vi "Calculate Attack Points.vi"(7 "Move Map":i32[][](array[numeric]), 8 "Team Index":i32, 9 "Max Atack Points":i32=4, 11 "Danger Map":i32[][](array[numeric])) -> (2 "Danger Columns Out":i32[](array[numeric]), 3 "Danger Rows Out":i32[](array[numeric]), 5 "Scores Out":i32[](array[numeric]))   [LabVIEW 2017, in "AntFarm_MB.lvclass"]
uses:
  AntFarm_MB.lvclass
panel:
  in  "Distance Threshold":dbl=2.9
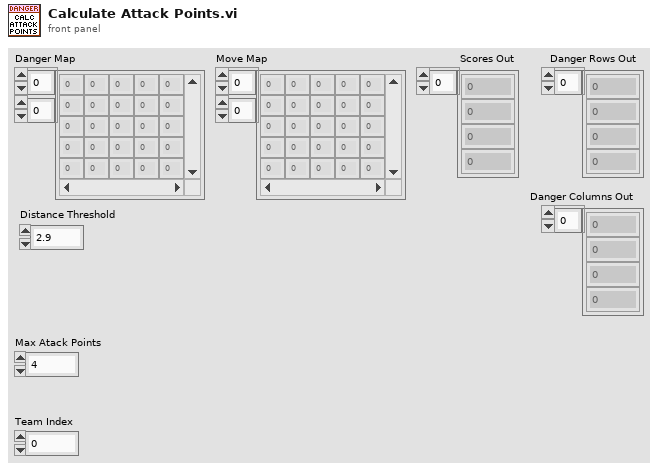
[diagram p1: front panel]
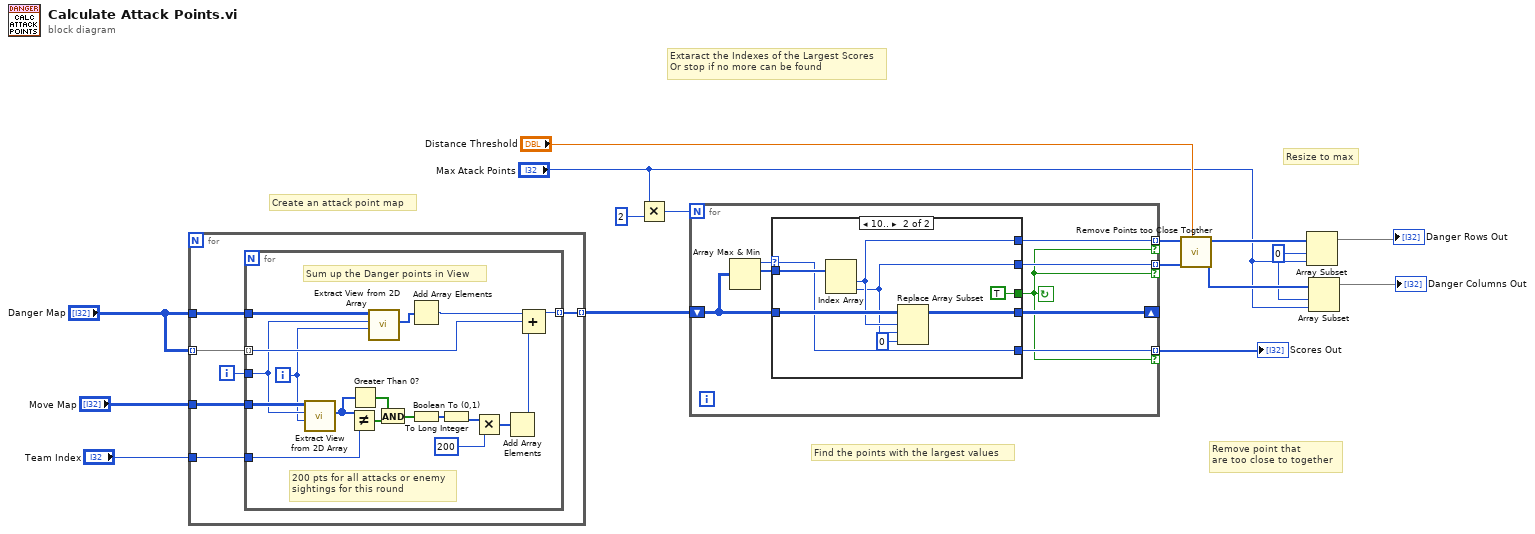
[diagram p0: block diagram]
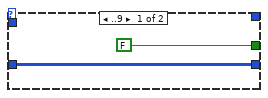
[diagram p2: hidden frame]
diagram:
  w1 = 0 ("index")
  # "Resize to max"
  # "Remove point that\nare too close to together"
  # "Find the points with the largest values"
  # "Create an attack point map"
  # "Extaract the Indexes of the Largest Scores\nOr stop if no more can be found"
  n1 = for {
    tunnel: "Danger Map" -> [w22] mode=indexing
    tunnel: "Danger Map" -> [w21]
    tunnel: [w19] -> w15 mode=indexing
    tunnel: "Move Map" -> [w18]
    tunnel: "Team Index" -> [w17]
    i -> [w20]
    n2 = for {
      tunnel: w22 -> [w37] mode=indexing
      tunnel: w21 -> [w40]
      tunnel: w20 -> [w30]
      tunnel: [w38] -> w19 mode=indexing
      tunnel: w18 -> [w33]
      tunnel: w17 -> [w35]
      i -> [w29]
      # "Sum up the Danger points in View"
      # "200 pts for all attacks or enemy\nsightings for this round"
      n3 = call "Extract View from 2D Array.vi"("Column"=w29, "Row"=w30, "Board Array"=w33) -> ("View Out"=w32:i32[])  [unwired: 7 in, 1 out]
      n4 = Not Equal?(x=w32, y=w35) -> (x != y?=w34:bool[])
      n5 = Greater Than 0?(x=w32) -> (x > 0?=w31:bool[])
      n6 = call "Extract View from 2D Array.vi"("Column"=w29, "Row"=w30, "Board Array"=w40) -> ("View Out"=w36:i32[])  [unwired: 7 in, 1 out]
      n7 = And(x=w31, y=w34) -> (x .and. y?=w28:bool[])
      n8 = Add Array Elements(numeric array=w36) -> (sum=w39:i32)
      n9 = Boolean To (0,1)(Boolean=w28) -> (0, 1=w27:i16[])
      n10 = To Long Integer(number=w27) -> (32bit integer=w26:i32[])
      n11 = Multiply(x=w26, y=200 ("Team Index 2")) -> (x*y=w24:i32[])
      n12 = Add Array Elements(numeric array=w24) -> (sum=w23:i32)
      n13 = Compound Arithmetic op=ADD(w39, w37, w23) -> (w38:i32)
    }
  }
  n14 = Multiply(x="Max Atack Points", y=2) -> (x*y=w11:i32)
  n15 = for {
    N: w11 -> [_]
    shift-right: [w46] -> _
    shift-left: w15 -> [w47]
    tunnel: [w44] -> w14 mode=indexing if=w41
    tunnel: [w43] -> w9 mode=indexing if=w41
    tunnel: [w42] -> w8 mode=indexing if=w41
    stop <- w41 continue-if-true
    n16 = Array Max & Min(array=w47) -> (max value=w48:i32, max index (indices)=w45:i32[])  [unwired: 2 out]
    n17 = case shown="10.." w48 {
      selector: w48 -> [_ w51]
      tunnel: w47 -> [w50 w56]
      tunnel: [w50 w55] -> w46
      tunnel: [FALSE TRUE] -> w41
      tunnel: w45 -> [_ w58]
      tunnel: [_ w51] -> w44
      tunnel: [_ w54] -> w43
      tunnel: [_ w53] -> w42
      frame ..9 {
      }
      frame 10.. {
        n18 = Index Array(array=w58) -> (element #1=w54:i32, element #2=w53:i32)  [unwired: 2 in]
        n19 = Replace Array Subset(array=w56, new element=0 ("new element/subarray"), index (row)=w54, index (col)=w53) -> (w55:i32[][])
      }
    }
  }
  "Scores Out" <- w14
  n20 = call "Remove Points too Close Togther.vi"("Distance Threshold"="Distance Threshold", "Columns"=w8, "Rows"=w9) -> ("Columns Out"=w6:i32[], "Rows Out"=w4:i32[])  [unwired: 7 in]
  n21 = Array Subset(array=w4, index=w1, length="Max Atack Points") -> (→"Danger Rows Out":i32[])
  n22 = Array Subset(array=w6, index=w1, length="Max Atack Points") -> (→"Danger Columns Out":i32[])
